vi "FA_StringToBoolean.vi"(0 "Input String":string="True", 1 "Error In":errorcluster) -> (14 "Boolean":bool=TRUE, 15 "Error Out":errorcluster)   [LabVIEW 2013, in "FA_ApplyRTEXE.lvlib"]
uses:
  FA_ApplyRTEXE.lvlib
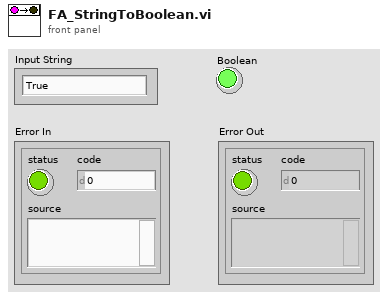
[diagram p1: front panel]
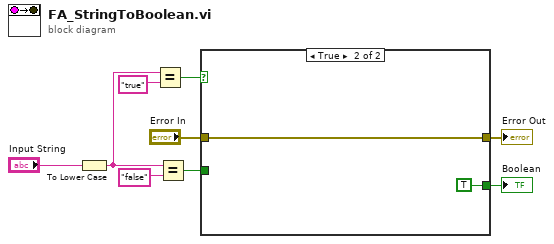
[diagram p0: block diagram]
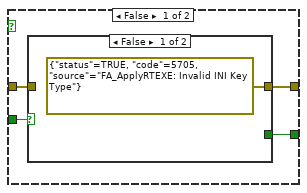
[diagram p2: hidden frame]
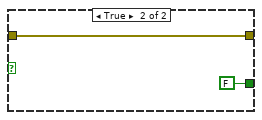
[diagram p3: hidden frame]
diagram:
  n1 = To Lower Case(string="Input String") -> (all lower case string=w6:string)
  n2 = Equal?(x=w6, y="true") -> (x = y?=w5:bool)
  n3 = Equal?(x=w6, y="false") -> (x = y?=w3:bool)
  n4 = case shown="True" w5 {
    tunnel: [w12 TRUE] -> w4
    tunnel: w3 -> [w13 _]
    tunnel: "Error In" -> [w11 w17]
    tunnel: [w10 w17] -> w1
    frame False {
      n5 = case shown="False" w13 {
        tunnel: [_ FALSE] -> w12
        tunnel: w11 -> [_ w15]
        tunnel: [errorcluster {"status"=TRUE, "code"=5705, "source"="FA_ApplyRTEXE: Invalid INI Key Type"} ("Error In") w15] -> w10
        frame False {
        }
        frame True {
        }
      }
    }
    frame True {
    }
  }
  "Boolean" <- w4
  "Error Out" <- w1
